vi "Build Simple Skeleton Data.vi"(8 "error in (no error)":errorcluster, 11 "data in":string) -> (0 "Kinect Outputs":T5, 1 "Skeleton Data":T6, 2 "NumPlayers":i8, 3 "Version String":string, 4 "Simple Joystick Info":T1(array[cluster]))   [LabVIEW 2012]
uses:
  <vilib>/addons/Kinect/SkeletonTrackState.ctl
  <vilib>/addons/Kinect/Vector4.ctl
  <vilib>/Rock Robotics/WPI/Joystick/WPI_JoystickDeviceDataRaw.ctl
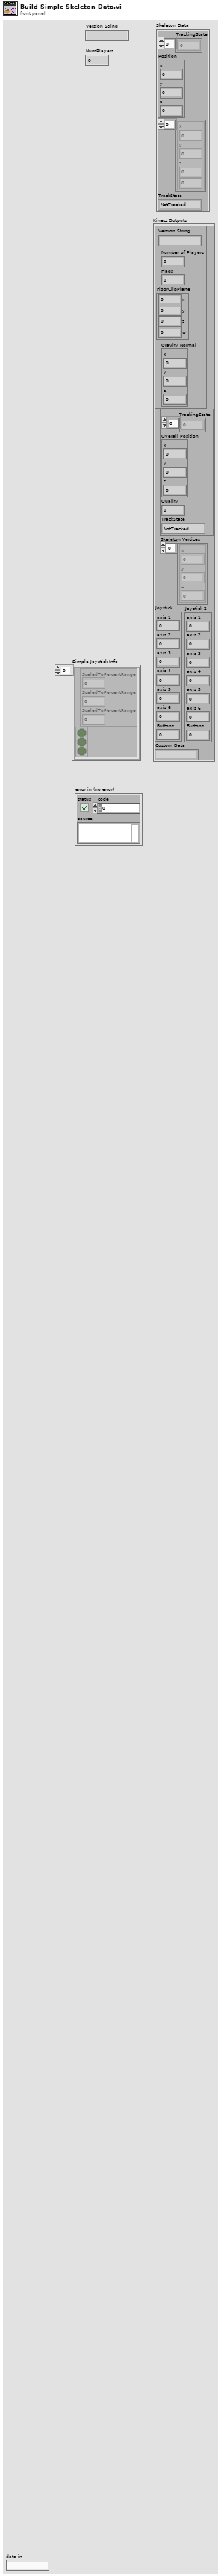
[diagram p1: front panel]
types:
  T1 = cluster{cluster{"ScaledToPercentRange":dbl, "ScaledToPercentRange":dbl, "ScaledToPercentRange":dbl}, cluster{bool, bool, bool}}[]
  T2 = typedef "Vector4.ctl" = cluster{"x":sgl, "y":sgl, "z":sgl, "w":sgl}
  T3 = typedef "SkeletonTrackState.ctl" = enum32{"NotTracked", "PositionOnly", "Tracked"}
  T4 = typedef "WPI_JoystickDeviceDataRaw.ctl" = cluster{"axis 1":i8, "axis 2":i8, "axis 3":i8, "axis 4":i8, "axis 5":i8, "axis 6":i8, "Buttons":u16}
  T5 = cluster{cluster{"Version String":string, "Number of Players":i8, "Flags":u32, "FloorClipPlane":T2, "Gravity Normal":cluster{"x":sgl, "y":sgl, "z":sgl}}, cluster{"TrackingState":u8[], "Overall Position":cluster{"x":sgl, "y":sgl, "z":sgl}, "Quality":u32, "TrackState":T3}, "Skeleton Vertices":cluster{"x":sgl, "y":sgl, "z":sgl}[], "Joystick":T4, "Joystick 2":T4, "Custom Data":string}
  T6 = cluster{"TrackingState":u8[], "Position":cluster{"x":sgl, "y":sgl, "z":sgl}, cluster{"x":sgl, "y":sgl, "z":sgl, sgl}[], "TrackState":T3}
  T7 = cluster{"size":u8, "tag":u8, "Version":cluster{"unsigned byte array[0]":u8, "unsigned byte array[1]":u8, "unsigned byte array[2]":u8, "unsigned byte array[3]":u8, "unsigned byte array[4]":u8, "unsigned byte array[5]":u8, "unsigned byte array[6]":u8, "unsigned byte array[7]":u8, "unsigned byte array[8]":u8, "unsigned byte array[9]":u8, "unsigned byte array[10]":u8}, "numPlayers":i8, "flags":u32, "floorClipPlane":T2, "Gravity Normal":cluster{"x":sgl, "y":sgl, "z":sgl}, "size":u8, "tag":u8, "Extra Data":cluster{"TrackingState":cluster{"TrackingState[0]":u8, "TrackingState[1]":u8, "TrackingState[2]":u8, "TrackingState[3]":u8, "TrackingState[4]":u8, "TrackingState[5]":u8, "TrackingState[6]":u8, "TrackingState[7]":u8, "TrackingState[8]":u8, "TrackingState[9]":u8, "TrackingState[10]":u8, "TrackingState[11]":u8, "TrackingState[12]":u8, "TrackingState[13]":u8, "TrackingState[14]":u8, "TrackingState[15]":u8, "TrackingState[16]":u8, "TrackingState[17]":u8, "TrackingState[18]":u8, "TrackingState[19]":u8}, "Position":cluster{"x":sgl, "y":sgl, "z":sgl}, "Quality":u32, "TrackState":T3}, "size":u8, "tag":u8, "Vertices":cluster{"Vertices[0]":cluster{"x":sgl, "y":sgl, "z":sgl}, "Vertices[1]":cluster{"x":sgl, "y":sgl, "z":sgl}, "Vertices[2]":cluster{"x":sgl, "y":sgl, "z":sgl}, "Vertices[3]":cluster{"x":sgl, "y":sgl, "z":sgl}, "Vertices[4]":cluster{"x":sgl, "y":sgl, "z":sgl}, "Vertices[5]":cluster{"x":sgl, "y":sgl, "z":sgl}, "Vertices[6]":cluster{"x":sgl, "y":sgl, "z":sgl}, "Vertices[7]":cluster{"x":sgl, "y":sgl, "z":sgl}, "Vertices[8]":cluster{"x":sgl, "y":sgl, "z":sgl}, "Vertices[9]":cluster{"x":sgl, "y":sgl, "z":sgl}, "Vertices[10]":cluster{"x":sgl, "y":sgl, "z":sgl}, "Vertices[11]":cluster{"x":sgl, "y":sgl, "z":sgl}, "Vertices[12]":cluster{"x":sgl, "y":sgl, "z":sgl}, "Vertices[13]":cluster{"x":sgl, "y":sgl, "z":sgl}, "Vertices[14]":cluster{"x":sgl, "y":sgl, "z":sgl}, "Vertices[15]":cluster{"x":sgl, "y":sgl, "z":sgl}, "Vertices[16]":cluster{"x":sgl, "y":sgl, "z":sgl}, "Vertices[17]":cluster{"x":sgl, "y":sgl, "z":sgl}, "Vertices[18]":cluster{"x":sgl, "y":sgl, "z":sgl}, "Vertices[19]":cluster{"x":sgl, "y":sgl, "z":sgl}}, "size":u8, "tag":u8, "Joystick":T4, "Joystick 2":T4, "size":u8, "tag":u8, "Custom Data":string}
  T8 = cluster{"unsigned byte array[0]":u8, "unsigned byte array[1]":u8, "unsigned byte array[2]":u8, "unsigned byte array[3]":u8, "unsigned byte array[4]":u8, "unsigned byte array[5]":u8, "unsigned byte array[6]":u8, "unsigned byte array[7]":u8, "unsigned byte array[8]":u8, "unsigned byte array[9]":u8, "unsigned byte array[10]":u8}
  T9 = cluster{"TrackingState[0]":u8, "TrackingState[1]":u8, "TrackingState[2]":u8, "TrackingState[3]":u8, "TrackingState[4]":u8, "TrackingState[5]":u8, "TrackingState[6]":u8, "TrackingState[7]":u8, "TrackingState[8]":u8, "TrackingState[9]":u8, "TrackingState[10]":u8, "TrackingState[11]":u8, "TrackingState[12]":u8, "TrackingState[13]":u8, "TrackingState[14]":u8, "TrackingState[15]":u8, "TrackingState[16]":u8, "TrackingState[17]":u8, "TrackingState[18]":u8, "TrackingState[19]":u8}
  T10 = cluster{"Vertices[0]":cluster{"x":sgl, "y":sgl, "z":sgl}, "Vertices[1]":cluster{"x":sgl, "y":sgl, "z":sgl}, "Vertices[2]":cluster{"x":sgl, "y":sgl, "z":sgl}, "Vertices[3]":cluster{"x":sgl, "y":sgl, "z":sgl}, "Vertices[4]":cluster{"x":sgl, "y":sgl, "z":sgl}, "Vertices[5]":cluster{"x":sgl, "y":sgl, "z":sgl}, "Vertices[6]":cluster{"x":sgl, "y":sgl, "z":sgl}, "Vertices[7]":cluster{"x":sgl, "y":sgl, "z":sgl}, "Vertices[8]":cluster{"x":sgl, "y":sgl, "z":sgl}, "Vertices[9]":cluster{"x":sgl, "y":sgl, "z":sgl}, "Vertices[10]":cluster{"x":sgl, "y":sgl, "z":sgl}, "Vertices[11]":cluster{"x":sgl, "y":sgl, "z":sgl}, "Vertices[12]":cluster{"x":sgl, "y":sgl, "z":sgl}, "Vertices[13]":cluster{"x":sgl, "y":sgl, "z":sgl}, "Vertices[14]":cluster{"x":sgl, "y":sgl, "z":sgl}, "Vertices[15]":cluster{"x":sgl, "y":sgl, "z":sgl}, "Vertices[16]":cluster{"x":sgl, "y":sgl, "z":sgl}, "Vertices[17]":cluster{"x":sgl, "y":sgl, "z":sgl}, "Vertices[18]":cluster{"x":sgl, "y":sgl, "z":sgl}, "Vertices[19]":cluster{"x":sgl, "y":sgl, "z":sgl}}
  T11 = cluster{"TrackingState":cluster{"TrackingState[0]":u8, "TrackingState[1]":u8, "TrackingState[2]":u8, "TrackingState[3]":u8, "TrackingState[4]":u8, "TrackingState[5]":u8, "TrackingState[6]":u8, "TrackingState[7]":u8, "TrackingState[8]":u8, "TrackingState[9]":u8, "TrackingState[10]":u8, "TrackingState[11]":u8, "TrackingState[12]":u8, "TrackingState[13]":u8, "TrackingState[14]":u8, "TrackingState[15]":u8, "TrackingState[16]":u8, "TrackingState[17]":u8, "TrackingState[18]":u8, "TrackingState[19]":u8}, "Position":cluster{"x":sgl, "y":sgl, "z":sgl}, "Quality":u32, "TrackState":T3}
  T12 = cluster{"ScaledToPercentRange":dbl, "ScaledToPercentRange":dbl, "ScaledToPercentRange":dbl}
  T13 = cluster{cluster{"ScaledToPercentRange":dbl, "ScaledToPercentRange":dbl, "ScaledToPercentRange":dbl}, cluster{bool, bool, bool}}
  T14 = cluster{"string":string, "numPlayers":i8, "flags":u32, "floorClipPlane":T2, "Gravity Normal":cluster{"x":sgl, "y":sgl, "z":sgl}}
  T15 = cluster{"TrackingState":u8[], "Position":cluster{"x":sgl, "y":sgl, "z":sgl}, "Quality":u32, "TrackState":T3}
  T16 = cluster{cluster{"string":string, "numPlayers":i8, "flags":u32, "floorClipPlane":T2, "Gravity Normal":cluster{"x":sgl, "y":sgl, "z":sgl}}, cluster{"TrackingState":u8[], "Position":cluster{"x":sgl, "y":sgl, "z":sgl}, "Quality":u32, "TrackState":T3}, "Vertices":cluster{"x":sgl, "y":sgl, "z":sgl}[], "Joystick":T4, "Joystick 2":T4, "Custom Data":string}
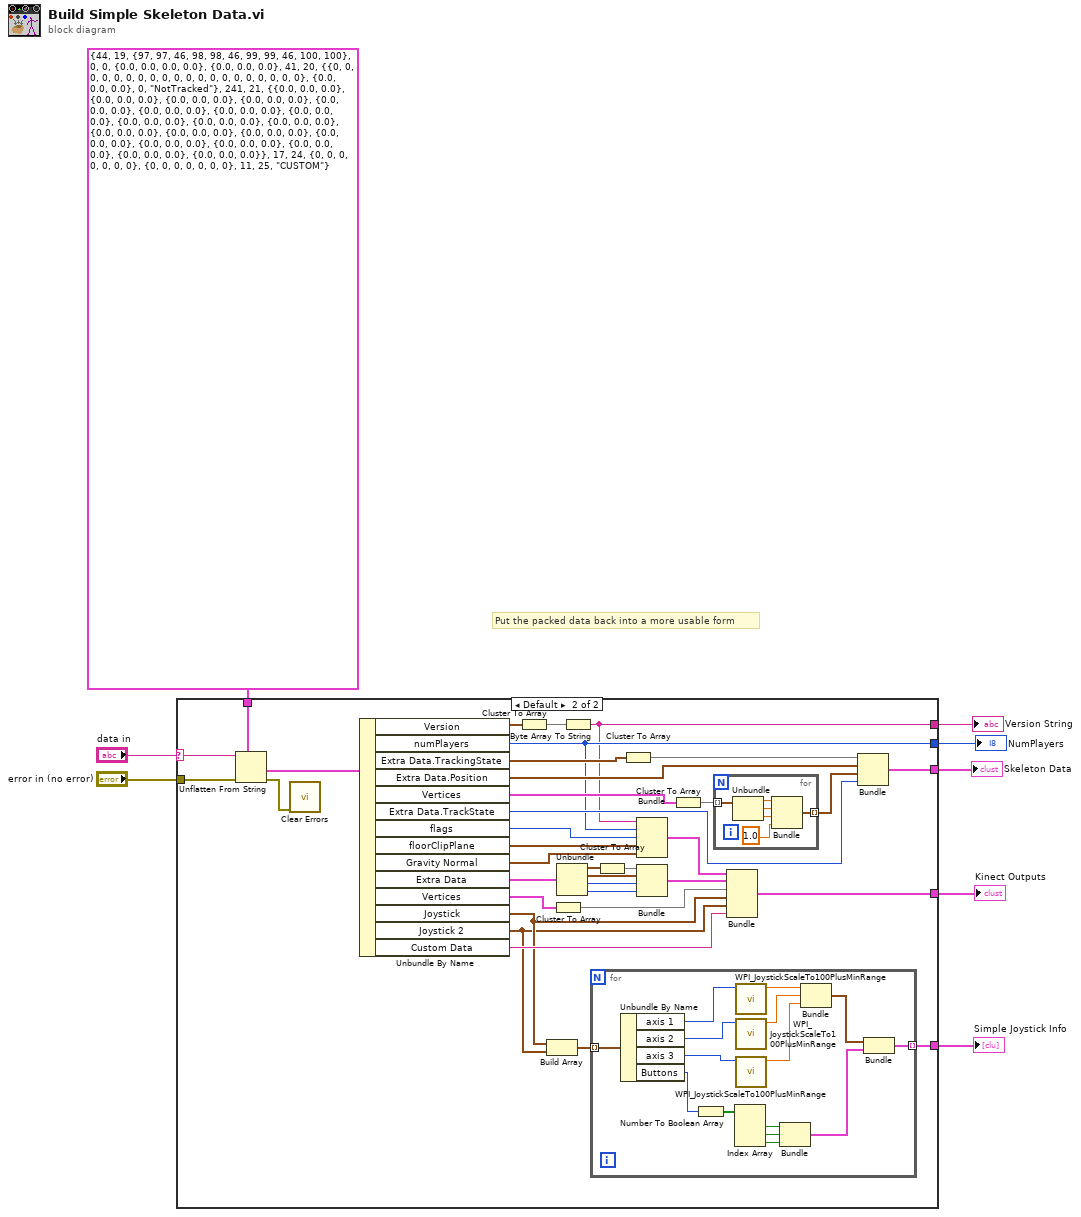
[diagram p0: block diagram]
diagram:
  # "Put the packed data back into a more usable form"
  n1 = case shown="Default" "data in" {
    selector: "data in" -> [_ w9]
    tunnel: [_ w38] -> w8
    tunnel: T7 {"size"=44, "tag"=19, "Version"={"unsigned byte array[0]"=97, "unsigned byte array[1]"=97, "unsigned byte array[2]"=46, "unsigned byte array[3]"=98, "unsigned byte array[4]"=98, "unsigned byte array[5]"=46, "unsigned byte array[6]"=99, "unsigned byte array[7]"=99, "unsigned byte array[8]"=46, "unsigned byte array[9]"=100, "unsigned byte array[10]"=100}, "numPlayers"=0, "flags"=0, "floorClipPlane"={"x"=0.0, "y"=0.0, "z"=0.0, "w"=0.0}, "Gravity Normal"={"x"=0.0, "y"=0.0, "z"=0.0}, "size"=41, "tag"=20, "Extra Data"={"TrackingState"={"TrackingState[0]"=0, "TrackingState[1]"=0, "TrackingState[2]"=0, "TrackingState[3]"=0, "TrackingState[4]"=0, "TrackingState[5]"=0, "TrackingState[6]"=0, "TrackingState[7]"=0, "TrackingState[8]"=0, "TrackingState[9]"=0, "TrackingState[10]"=0, "TrackingState[11]"=0, "TrackingState[12]"=0, "TrackingState[13]"=0, "TrackingState[14]"=0, "TrackingState[15]"=0, "TrackingState[16]"=0, "TrackingState[17]"=0, "TrackingState[18]"=0, "TrackingState[19]"=0}, "Position"={"x"=0.0, "y"=0.0, "z"=0.0}, "Quality"=0, "TrackState"=enum."NotTracked"}, "size"=241, "tag"=21, "Vertices"={"Vertices[0]"={"x"=0.0, "y"=0.0, "z"=0.0}, "Vertices[1]"={"x"=0.0, "y"=0.0, "z"=0.0}, "Vertices[2]"={"x"=0.0, "y"=0.0, "z"=0.0}, "Vertices[3]"={"x"=0.0, "y"=0.0, "z"=0.0}, "Vertices[4]"={"x"=0.0, "y"=0.0, "z"=0.0}, "Vertices[5]"={"x"=0.0, "y"=0.0, "z"=0.0}, "Vertices[6]"={"x"=0.0, "y"=0.0, "z"=0.0}, "Vertices[7]"={"x"=0.0, "y"=0.0, "z"=0.0}, "Vertices[8]"={"x"=0.0, "y"=0.0, "z"=0.0}, "Vertices[9]"={"x"=0.0, "y"=0.0, "z"=0.0}, "Vertices[10]"={"x"=0.0, "y"=0.0, "z"=0.0}, "Vertices[11]"={"x"=0.0, "y"=0.0, "z"=0.0}, "Vertices[12]"={"x"=0.0, "y"=0.0, "z"=0.0}, "Vertices[13]"={"x"=0.0, "y"=0.0, "z"=0.0}, "Vertices[14]"={"x"=0.0, "y"=0.0, "z"=0.0}, "Vertices[15]"={"x"=0.0, "y"=0.0, "z"=0.0}, "Vertices[16]"={"x"=0.0, "y"=0.0, "z"=0.0}, "Vertices[17]"={"x"=0.0, "y"=0.0, "z"=0.0}, "Vertices[18]"={"x"=0.0, "y"=0.0, "z"=0.0}, "Vertices[19]"={"x"=0.0, "y"=0.0, "z"=0.0}}, "size"=17, "tag"=24, "Joystick"={"axis 1"=0, "axis 2"=0, "axis 3"=0, "axis 4"=0, "axis 5"=0, "axis 6"=0, "Buttons"=0}, "Joystick 2"={"axis 1"=0, "axis 2"=0, "axis 3"=0, "axis 4"=0, "axis 5"=0, "axis 6"=0, "Buttons"=0}, "size"=11, "tag"=25, "Custom Data"="CUSTOM"} ("output data") -> [_ w34]
    tunnel: [_ w31] -> w6
    tunnel: [_ w17] -> w5
    tunnel: [_ w16] -> w4
    tunnel: [_ w11] -> w3
    tunnel: "error in (no error)" -> [_ w10]
    frame "" {
    }
    frame Default {
      n2 = Unflatten From String(type=w34, binary string=w9, error in (no error)=w10) -> (value=w35:T7, error out=w33:errorcluster)  [unwired: 3 out]
      n3 = call <vilib>:"Clear Errors.vi"("error in (no error)"=w33) -> ()  [unwired: 6 in, 1 out]
      n4 = Unbundle By Name(w35) -> ("Version"=w32:T8, "numPlayers"=w31:i8, "Extra Data.TrackingState"=w37:T9, "Extra Data.Position"=w43:cluster{"x":sgl, "y":sgl, "z":sgl}, "Vertices"=w42:T10, "Extra Data.TrackState"=w44:T3, "flags"=w30:u32, "floorClipPlane"=w29:T2, "Gravity Normal"=w28:cluster{"x":sgl, "y":sgl, "z":sgl}, "Extra Data"=w26:T11, "Vertices"=w19:T10, "Joystick"=w14:T4, "Joystick 2"=w12:T4, "Custom Data"=w15:string)
      n5 = Cluster To Array(cluster=w32) -> (array=w36:u8[])
      n6 = Build Array(w14, w12) -> (w13:T4[])
      n7 = Cluster To Array(cluster=w19) -> (array=w18:cluster{"x":sgl, "y":sgl, "z":sgl}[])
      n8 = Unbundle(w26) -> ("TrackingState"=w25:T9, "Position"=w23:cluster{"x":sgl, "y":sgl, "z":sgl}, "Quality"=w22:u32, "TrackState"=w21:T3)
      n9 = Byte Array To String(unsigned byte array=w36) -> (string=w16:string)
      n10 = for {
        tunnel: w13 -> [w59] mode=indexing
        tunnel: [w45] -> w11 mode=indexing
        n11 = Unbundle By Name(w59) -> ("axis 1"=w53:i8, "axis 2"=w51:i8, "axis 3"=w50:i8, "Buttons"=w57:u16)
        n12 = Number To Boolean Array(number=w57) -> (Boolean array=w58:bool[])
        n13 = Index Array(array=w58) -> (element #1=w54:bool, element #2=w55:bool, element #3=w56:bool)  [unwired: 3 in]
        n14 = call <vilib>:"WPI_JoystickScaleTo100PlusMinRange.vi"("RawValue"=w53) -> ("ScaledToPercentRange"=w52:dbl)  [unwired: 1 in, 9 out]
        n15 = call <vilib>:"WPI_JoystickScaleTo100PlusMinRange.vi"("RawValue"=w51) -> ("ScaledToPercentRange"=w49:dbl)  [unwired: 1 in, 9 out]
        n16 = call <vilib>:"WPI_JoystickScaleTo100PlusMinRange.vi"("RawValue"=w50) -> ("ScaledToPercentRange"=w48:dbl)  [unwired: 1 in, 9 out]
        n17 = Bundle(w54, w55, w56) -> (w46:cluster{bool, bool, bool})  [unwired: 1 in]
        n18 = Bundle("ScaledToPercentRange"=w52, "ScaledToPercentRange"=w49, "ScaledToPercentRange"=w48) -> (w47:T12)  [unwired: 1 in]
        n19 = Bundle(w47, w46) -> (w45:T13)  [unwired: 1 in]
      }
      n20 = Cluster To Array(cluster=w25) -> (array=w24:u8[])
      n21 = Cluster To Array(cluster=w37) -> (array=w39:u8[])
      n22 = Bundle("string"=w16, "numPlayers"=w31, "flags"=w30, "floorClipPlane"=w29, "Gravity Normal"=w28) -> (w27:T14)  [unwired: 1 in]
      n23 = Bundle("TrackingState"=w24, "Position"=w23, "Quality"=w22, "TrackState"=w21) -> (w20:T15)  [unwired: 1 in]
      n24 = Cluster To Array(cluster=w42) -> (array=w40:cluster{"x":sgl, "y":sgl, "z":sgl}[])
      n25 = for {
        tunnel: w40 -> [w65] mode=indexing
        tunnel: [w60] -> w41 mode=indexing
        n26 = Unbundle(w65) -> ("x"=w61:sgl, "y"=w62:sgl, "z"=w63:sgl)
        n27 = Bundle("x"=w61, "y"=w62, "z"=w63, sgl 1.0) -> (w60:cluster{"x":sgl, "y":sgl, "z":sgl, sgl})  [unwired: 1 in]
      }
      n28 = Bundle(w27, w20, "Vertices"=w18, "Joystick"=w14, "Joystick 2"=w12, "Custom Data"=w15) -> (w17:T16)  [unwired: 1 in]
      n29 = Bundle("TrackingState"=w39, "Position"=w43, w41, "TrackState"=w44) -> (w38:T6)  [unwired: 1 in]
    }
  }
  "Skeleton Data" <- w8
  "NumPlayers" <- w6
  "Version String" <- w4
  "Kinect Outputs" <- w5
  "Simple Joystick Info" <- w3
